vi "ConvertStrings(Hex to Normal).vi"(3 "Hex String":string="H\f\u0000D\u0014\u0014") -> (1 "Normal String":string)   [LabVIEW 2013]
panel:
  # "RE-ENTRANT"
  # "SUB-ROUTINE"
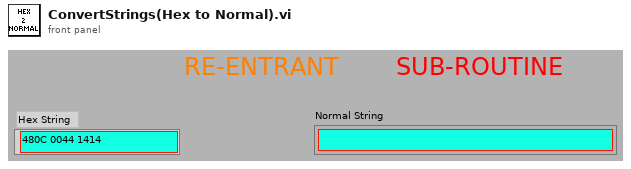
[diagram p1: front panel]
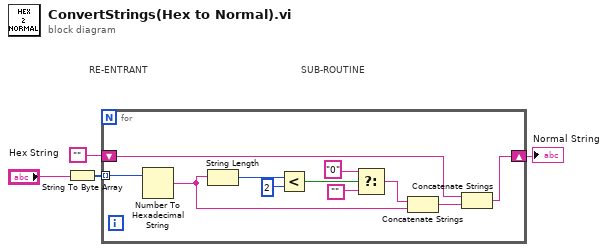
[diagram p0: block diagram]
diagram:
  # "SUB-ROUTINE"
  # "RE-ENTRANT"
  n1 = String To Byte Array(string="Hex String") -> (unsigned byte array=w3:u8[])
  n2 = for {
    shift-right: [w15] -> w1
    shift-left: "" -> [w8]
    tunnel: w3 -> [w5] mode=indexing
    n3 = Number To Hexadecimal String(2:w5) -> (0:w7:string)  [unwired: 1 in]
    n4 = String Length(string=w7) -> (length=w14:i32)
    n5 = Less?(x=w14, y=2) -> (x < y?=w12:bool)
    n6 = Select(t="0", s=w12, f="") -> (s? t:f=w9:string)
    n7 = Concatenate Strings(w9, w7) -> (w6:string)
    n8 = Concatenate Strings(w8, w6) -> (w15:string)
  }
  "Normal String" <- w1
